vi "Auto Set Shooter RPM.vi"() -> (2 "READY!":bool, 3 "Vbus Out":dbl)   [LabVIEW 2012]
uses:
  BotStatus.vi
  <vilib>/express/express arith-compare/Formula/XNode/ExpressFormulaBlockNode.xnode
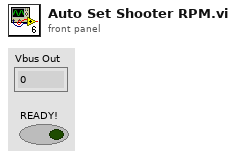
[diagram p1: front panel]
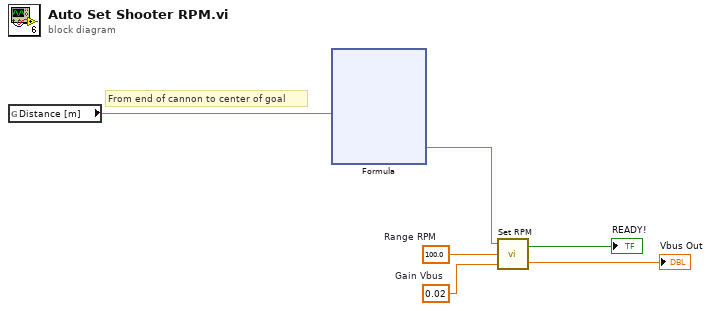
[diagram p0: block diagram]
diagram:
  w5 = 0.02  # Gain Vbus
  w6 = 100.0  # Range RPM
  # "From end of cannon to center of goal"
  n1 = global read "BotStatus.vi" "Distance [m]"() -> (w2:dbl)
  n2 = xnode "Formula"("D"=w2) -> ("Result"=w1:dbl)  [unwired: 2 in, 1 out]
  n3 = call "Set RPM.vi"("Gain Vbus"=w5, "Range RPM"=w6, "Set Point RPM"=w1) -> ("Vbus Out"=→"Vbus Out":dbl, "READY!"=→"READY!":bool)
